vi "Test Process Stop without Start.vi"(8 "error in (no error)":errorcluster, 11 "Process Test In":refnum<class "Process Dev Test.lvclass">) -> (0 "error out":errorcluster, 3 "Process Test Out":refnum<class "Process Dev Test.lvclass">)   [LabVIEW 2020, in "Process Dev Test.lvclass"]
uses:
  Process Dev Test.lvclass
  C:/Git/astemes-triarc-framework/source/TF Test Suite/Base Class Test/Base Test.lvclass
  C:/Program Files (x86)/National Instruments/LabVIEW 2020/vi.lib/Astemes/LUnit/Test Case.lvclass
  source/Framework/Process/Process.lvclass
  source/Framework Test Suite/Base Class Test/Base Test.lvclass/Base Test.ctl
  source/Framework/Process/Process.lvclass/Process.ctl
  <vilib>/Astemes/LUnit/Test Case.lvclass/Test Case.ctl
  <vilib>/Astemes/LUnit/LUnit Assertion Result.lvclass/LUnit Assertion Result.ctl
  <vilib>/Astemes/LUnit/LUnit Test Case Result.lvclass/LUnit Test Case Result.ctl
  <vilib>/Astemes/LUnit/LUnit Method Result.lvclass/LUnit Method Result.ctl
  source/Framework/Process/Private/SubVIs/Wait for finish.vi
  source/Framework/Process/Protected/Messaging/Enqueue Message.vi
  source/Framework/Process/Private/SubVIs/Set Lifecycle State.vi
  source/Framework/Process/Public/Lifecycle/Get Lifecycle State.vi
  <vilib>/Astemes/LUnit/Palette/Fail.vi
  <vilib>/Astemes/LUnit/Palette/Pass.vi
  <vilib>/Astemes/LUnit/Set Assertion Type.vi
  source/Framework/Process/Private/SubVIs/Handle Debug Data.vi
  <vilib>/Utility/error.llb/Clear Errors.vi
  <vilib>/Astemes/LUnit/Add test result.vi
  <vilib>/Astemes/LUnit/LUnit Write Passed.vi
  <vilib>/Astemes/LUnit/LUnit Write Message.vi
  <vilib>/Astemes/LUnit/LUnit Write Description.vi
  <vilib>/Astemes/LUnit/LUnit Write Assertion Type.vi
  source/Framework/Logging/Log Debug.vi
  <vilib>/AdvancedString/1D String Array to Delimited String.vi
  <vilib>/Utility/High Resolution Relative Seconds.vi
  <vilib>/Astemes/LUnit/LUnit Record Assertion Result.vi
  <vilib>/Astemes/LUnit/LUnit Aggregate Assertion Results.vi
  <vilib>/Astemes/LUnit/Assertion Result/LUnit Read Status.vi
  <vilib>/Astemes/LUnit/LUnit Read Message.vi
  <vilib>/Astemes/LUnit/LUnit Read Description.vi
  <vilib>/Astemes/LUnit/Method Result/LUnit Merge Status.vi
  <vilib>/Astemes/LUnit/LUnit Concatenate result strings.vi
  <vilib>/Utility/error.llb/Error Cluster From Error Code.vi
  source/Framework/Process/Public/Read Name.vi
  source/Framework/Base/Base.lvclass
  <vilib>/Astemes/LUnit/LUnit Assertion Result.lvclass
  <vilib>/Astemes/LUnit/Test Case.lvclass
  source/Framework Test Suite/Base Class Test/Base Test.lvclass
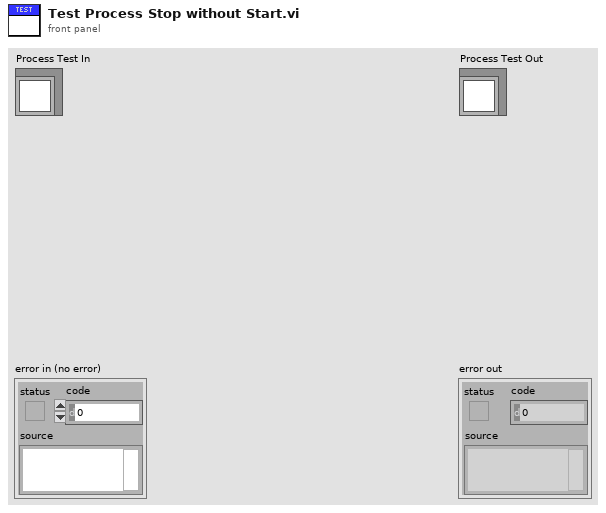
[diagram p1: front panel]
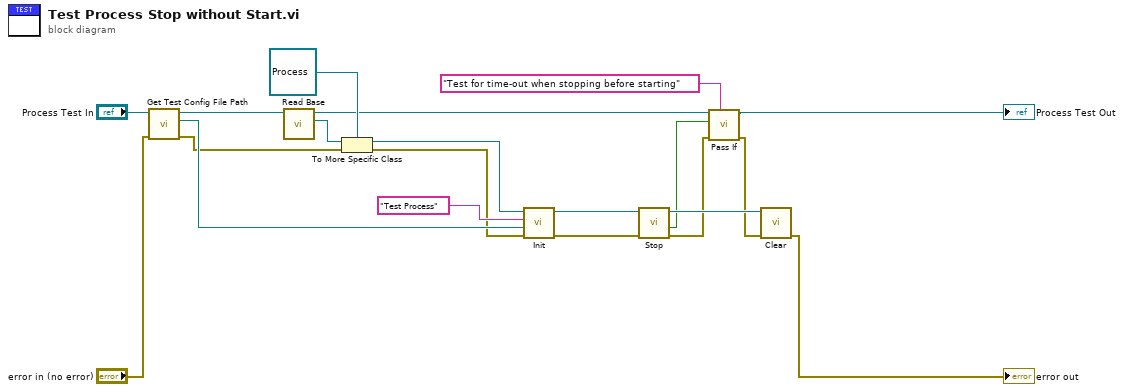
[diagram p0: block diagram]
diagram:
  n1 = call "Get Test Config File Path.vi"("error in (no error)"="error in (no error)", "Process Test In"="Process Test In") -> ("error out"=w4:errorcluster, "Test config path"=w9:path, "Process Test Out"=w6:refnum<class "Process Dev Test.lvclass">)  [unwired: 7 in]
  n2 = call "Read Base.vi"("Base Class Test In"=w6) -> ("Base.lvclass"=w7:refnum<class "Base.lvclass">, "Base Class Test Out"=w5:refnum<class "Process Dev Test.lvclass">)  [unwired: 8 in, 1 out]
  n3 = To More Specific Class(target class=refnum<class "Process.lvclass"> refnum ("Process.lvclass"), reference=w7, error in=w4) -> (specific class reference=w2:refnum<class "Process.lvclass">, error out=w3:errorcluster)
  n4 = call-dynamic "Init.vi"("error in (no error)"=w3, "Config File Path"=w9, "Name"="Test Process", "Process In"=w2) -> ("error out"=w12:errorcluster, "Process Out"=w15:refnum<class "Process.lvclass">)  [unwired: 6 in]
  n5 = call "Stop.vi"("error in (no error)"=w12, "Process In"=w15) -> ("error out"=w18:errorcluster, "timed out?"=w19:bool, "Process Out"=w20:refnum<class "Process.lvclass">)  [unwired: 7 in]
  n6 = call <vilib>:"Pass If.vi"("Description"="Test for time-out when stopping before starting" ("custom report message (\"\")"), "error in (no error)"=w18, "Pass?"=w19, "LUnit Test Case In"=w5) -> ("error out"=w14:errorcluster, "LUnit Test Case Out"=→"Process Test Out":refnum<class "Process Dev Test.lvclass">)  [unwired: 6 in]
  n7 = call-dynamic "Clear.vi"("error in (no error)"=w14, "Process In"=w20) -> ("error out"=→"error out":errorcluster)  [unwired: 9 in]
